vi "preScanHoldTime.vi"(8 "error in (no error)":errorcluster, 11 "PeriodicWave in":refnum<class "PeriodicWave.lvclass">) -> (0 "error out":errorcluster, 2 "PrescanHold?":bool=TRUE, 3 "PeriodicWave out":refnum<class "PeriodicWave.lvclass">)   [LabVIEW 2015, in "PeriodicWave.lvclass"]
uses:
  PeriodicWave.lvclass
  PeriodicWave.lvclass/PeriodicWave.ctl
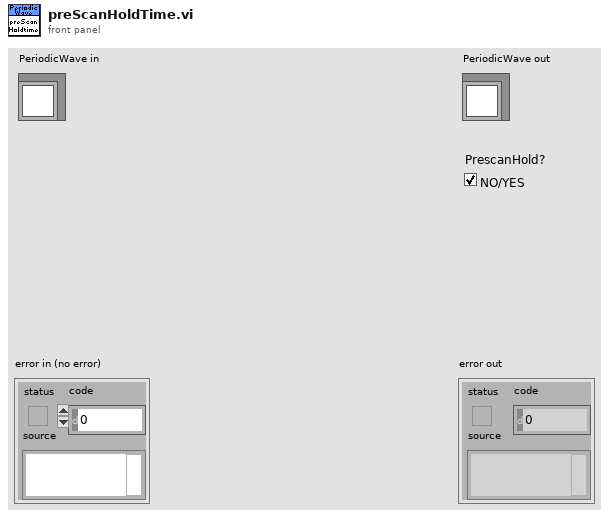
[diagram p1: front panel]
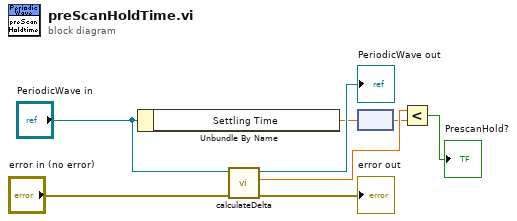
[diagram p0: block diagram]
diagram:
  n1 = Unbundle By Name("PeriodicWave in") -> ("Settling Time"=w5:dbl[unit])
  n2 = call "calculateDelta.vi"("error in (no error)"="error in (no error)", "PeriodicWave in"="PeriodicWave in") -> ("error out"=→"error out":errorcluster, "Delta Timestamp"=w6:dbl, "PeriodicWave out"=→"PeriodicWave out":refnum<class "PeriodicWave.lvclass">)  [unwired: 7 in]
  n3 = node(w5) -> (w4:dbl)
  n4 = Less?(x=w6, y=w4) -> (x < y?=→"PrescanHold?":bool)
